vi "8 PulseGenerations.vi"(2 "PulseGen Packets":u64[](array[numeric])=[0, 0, 0, 0, 0, 0, 0, 0], 4 "8 PulseGen Chs":T1={"DO0"="Connector0/DIO4", "DO1"="Connector0/DIO5", "DO2"="Connector0/DIO6", "DO3"="Connector0/DIO7", "DO4"="Connector0/DIO12", "DO5"="Connector0/DIO13", "DO6"="Connector0/DIO14", "DO7"="Connector0/DIO15"}) -> ()   [LabVIEW 2010]
uses:
  <vilib>/eio/EIONode/EIONode.xnode
  <vilib>/rvi/eio/nirviEIOImplementation/nirviEIOImplementation.xnode
  <vilib>/rvi/eio/common/nirviEmuClasses.ctl
  <vilib>/rvi/eio/common/nirviEmuTemplateMethod_noerrors.vi
  <vilib>/NI Veristand/FPGA/NI_VS FPGA Support.lvlib
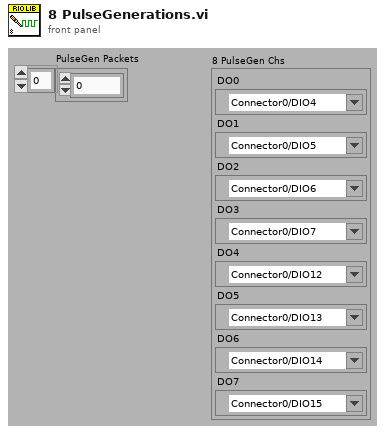
[diagram p1: front panel]
types:
  T1 = cluster{"DO0":refnum<k21>, "DO1":refnum<k21>, "DO2":refnum<k21>, "DO3":refnum<k21>, "DO4":refnum<k21>, "DO5":refnum<k21>, "DO6":refnum<k21>, "DO7":refnum<k21>}
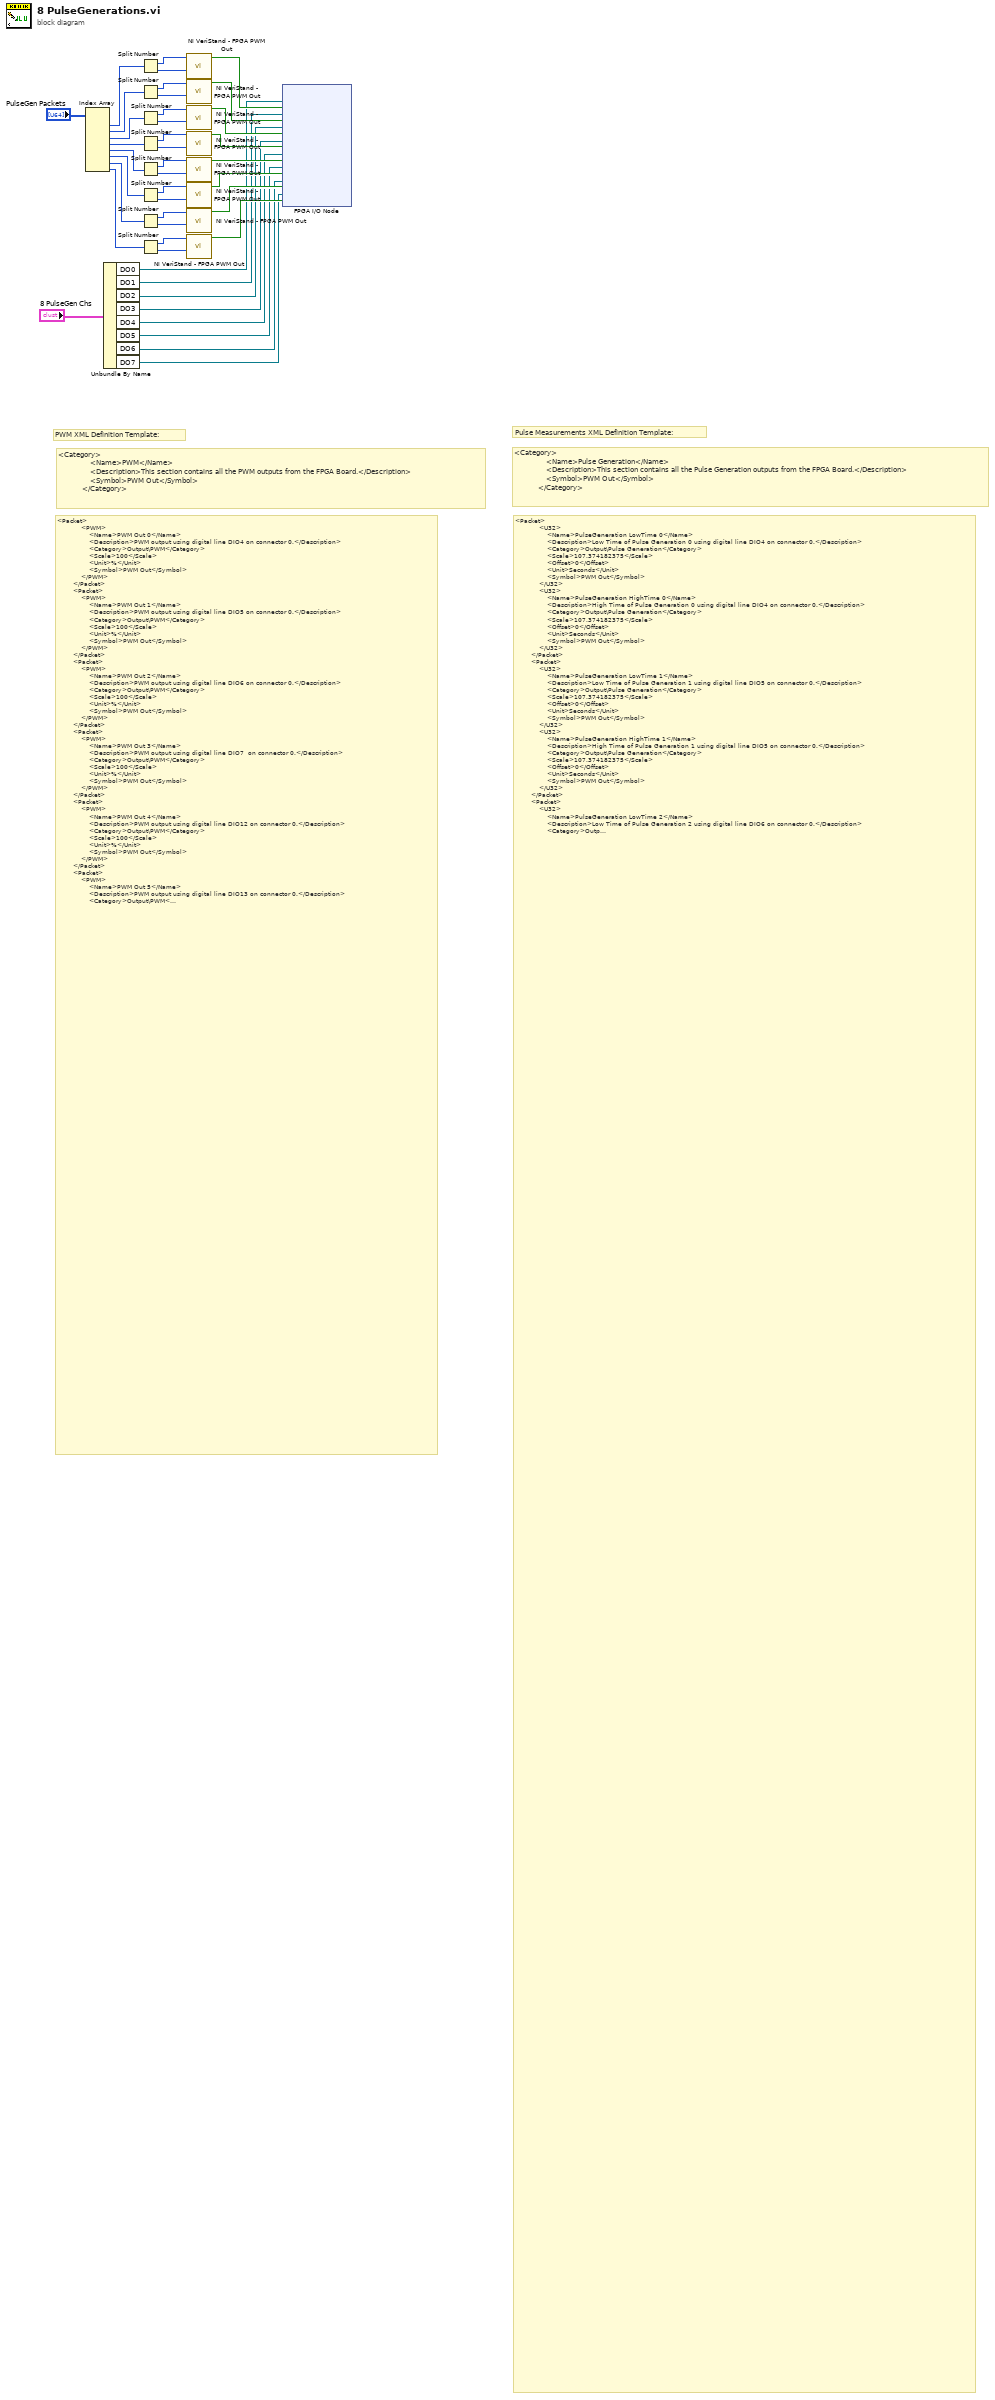
[diagram p0: block diagram]
diagram:
  # "<Category>\n                <Name>Pulse Generation</Name>\n                <Description>This section contains all the Pulse Generation outputs from the FPGA Board.</Description>\n                <Symbol>PWM Out</Symbol>\n            </Category>"
  # "<Category>\n                <Name>PWM</Name>\n                <Description>This section contains all the PWM outputs from the FPGA Board.</Description>\n                <Symbol>PWM Out</Symbol>\n            </Category>"
  # "Pulse Measurements XML Definition Template:"
  # "<Packet>\n            <U32>\n                <Name>PulseGeneration LowTime 0</Name>\n                <Description>Low Time of Pulse Generation 0 using digital line DIO4 on connector 0.</Description>\n                <Category>Output\\Pulse Generation</Category>\n                <Scale>107.374182375</Scale>\n                <Offset>0</Offset>\n                <Unit>Seconds</Unit>\n                <Symbol>PWM Out</Symbol>\n            </U32>\n            <U32>\n                <Name>PulseGeneration HighTime 0</Name>\n                <Description>High Time of Pulse Generation 0 using digital line DIO4 on connector 0.</Description>\n                <Category>Output\\Pulse Generation</Category>\n                <Scale>107.374182375</Scale>\n                <Offset>0</Offset>\n                <Unit>Seconds</Unit>\n                <Symbol>PWM Out</Symbol>\n            </U32>\n        </Packet>\n        <Packet>\n            <U32>\n                <Name>PulseGeneration LowTime 1</Name>\n                <Description>Low Time of Pulse Generation 1 using digital line DIO5 on connector 0.</Description>\n                <Category>Output\\Pulse Generation</Category>\n                <Scale>107.374182375</Scale>\n                <Offset>0</Offset>\n                <Unit>Seconds</Unit>\n                <Symbol>PWM Out</Symbol>\n            </U32>\n            <U32>\n                <Name>PulseGeneration HighTime 1</Name>\n                <Description>High Time of Pulse Generation 1 using digital line DIO5 on connector 0.</Description>\n                <Category>Output\\Pulse Generation</Category>\n                <Scale>107.374182375</Scale>\n                <Offset>0</Offset>\n                <Unit>Seconds</Unit>\n                <Symbol>PWM Out</Symbol>\n            </U32>\n        </Packet>\n        <Packet>\n            <U32>\n                <Name>PulseGeneration LowTime 2</Name>\n                <Description>Low Time of Pulse Generation 2 using digital line DIO6 on connector 0.</Description>\n                <Category>Output\\Pulse Generation</Category>\n                <Scale>107.374182375</Scale>\n                <Offset>0</Offset>\n                <Unit>Seconds</Unit>\n                <Symbol>PWM Out</Symbol>\n            </U32>\n            <U32>\n                <Name>PulseGeneration HighTime 2</Name>\n                <Description>High Time of Pulse Generation 2 using digital line DIO6 on connector 0.</Description>\n                <Category>Output\\Pulse Generation</Category>\n                <Scale>107.374182375</Scale>\n                <Offset>0</Offset>\n                <Unit>Seconds</Unit>\n                <Symbol>PWM Out</Symbol>\n            </U32>\n        </Packet>\n        <Packet>\n            <U32>\n                <Name>PulseGeneration LowTime 3</Name>\n                <Description>Low Time of Pulse Generation 3 using digital line DIO7 on connector 0.</Description>\n                <Category>Output\\Pulse Generation</Category>\n                <Scale>107.374182375</Scale>\n                <Offset>0</Offset>\n                <Unit>Seconds</Unit>\n                <Symbol>PWM Out</Symbol>\n            </U32>\n            <U32>\n                <Name>PulseGeneration HighTime 3</Name>\n                <Description>High Time of Pulse Generation 3 using digital line DIO7 on connector 0.</Description>\n                <Category>Output\\Pulse Generation</Category>\n                <Scale>107.374182375</Scale>\n                <Offset>0</Offset>\n                <Unit>Seconds</Unit>\n                <Symbol>PWM Out</Symbol>\n            </U32>\n        </Packet>\n        <Packet>\n            <U32>\n                <Name>PulseGeneration LowTime 4</Name>\n                <Description>Low Time of Pulse Generation 4 using digital line DIO12 on connector 0.</Description>\n                <Category>Output\\Pulse Generation</Category>\n                <Scale>107.374182375</Scale>\n                <Offset>0</Offset>\n                <Unit>Seconds</Unit>\n                <Symbol>PWM Out</Symbol>\n            </U32>\n            <U32>\n                <Name>PulseGeneration HighTime 4</Name>\n                <Description>High Time of Pulse Generation 4 using digital line DIO12 on connector 0.</Description>\n                <Category>Output\\Pulse Generation</Category>\n                <Scale>107.374182375</Scale>\n                <Offset>0</Offset>\n                <Unit>Seconds</Unit>\n                <Symbol>PWM Out</Symbol>\n            </U32>\n        </Packet>\n        <Packet>\n            <U32>\n                <Name>PulseGeneration LowTime 5</Name>\n                <Description>Low Time of Pulse Generation 5 using digital line DIO13 on connector 0.</Description>\n                <Category>Output\\Pulse Generation</Category>\n                <Scale>107.374182375</Scale>\n                <Offset>0</Offset>\n                <Unit>Seconds</Unit>\n                <Symbol>PWM Out</Symbol>\n            </U32>\n            <U32>\n                <Name>PulseGeneration HighTime 5</Name>\n                <Description>High Time of Pulse Generation 5 using digital line DIO13 on connector 0.</Description>\n                <Category>Output\\Pulse Generation</Category>\n                <Scale>107.374182375</Scale>\n                <Offset>0</Offset>\n                <Unit>Seconds</Unit>\n                <Symbol>PWM Out</Symbol>\n            </U32>\n        </Packet>\n        <Packet>\n            <U32>\n                <Name>PulseGeneration LowTime 6</Name>\n                <Description>Low Time of Pulse Generation 6 using digital line DIO14 on connector 0.</Description>\n                <Category>Output\\Pulse Generation</Category>\n                <Scale>107.374182375</Scale>\n                <Offset>0</Offset>\n                <Unit>Seconds</Unit>\n                <Symbol>PWM Out</Symbol>\n            </U32>\n            <U32>\n                <Name>PulseGeneration HighTime 6</Name>\n                <Description>High Time of Pulse Generation 6 using digital line DIO14 on connector 0.</Description>\n                <Category>Output\\Pulse Generation</Category>\n                <Scale>107.374182375</Scale>\n                <Offset>0</Offset>\n                <Unit>Seconds</Unit>\n                <Symbol>PWM Out</Symbol>\n            </U32>\n        </Packet>\n        <Packet>\n            <U32>\n                <Name>PulseGeneration LowTime 7</Name>\n                <Description>Low Time of Pulse Generation 7 using digital line DIO15 on connector 0.</Description>\n                <Category>Output\\Pulse Generation</Category>\n                <Scale>107.374182375</Scale>\n                <Offset>0</Offset>\n                <Unit>Seconds</Unit>\n                <Symbol>PWM Out</Symbol>\n            </U32>\n            <U32>\n                <Name>PulseGeneration HighTime 7</Name>\n                <Description>High Time of Pulse Generation 7 using digital line DIO15 on connector 0.</Description>\n                <Category>Output\\Pulse Generation</Category>\n                <Scale>107.374182375</Scale>\n                <Offset>0</Offset>\n                <Unit>Seconds</Unit>\n                <Symbol>PWM Out</Symbol>\n            </U32>\n        </Packet>"
  # "PWM XML Definition Template:"
  # "<Packet>\n            <PWM>\n                <Name>PWM Out 0</Name>\n                <Description>PWM output using digital line DIO4 on connector 0.</Description>\n                <Category>Output\\PWM</Category>\n                <Scale>100</Scale>\n                <Unit>%</Unit>\n                <Symbol>PWM Out</Symbol>\n            </PWM>\n        </Packet>\n        <Packet>\n            <PWM>\n                <Name>PWM Out 1</Name>\n                <Description>PWM output using digital line DIO5 on connector 0.</Description>\n                <Category>Output\\PWM</Category>\n                <Scale>100</Scale>\n                <Unit>%</Unit>\n                <Symbol>PWM Out</Symbol>\n            </PWM>\n        </Packet>\n        <Packet>\n            <PWM>\n                <Name>PWM Out 2</Name>\n                <Description>PWM output using digital line DIO6 on connector 0.</Description>\n                <Category>Output\\PWM</Category>\n                <Scale>100</Scale>\n                <Unit>%</Unit>\n                <Symbol>PWM Out</Symbol>\n            </PWM>\n        </Packet>\n        <Packet>\n            <PWM>\n                <Name>PWM Out 3</Name>\n                <Description>PWM output using digital line DIO7  on connector 0.</Description>\n                <Category>Output\\PWM</Category>\n                <Scale>100</Scale>\n                <Unit>%</Unit>\n                <Symbol>PWM Out</Symbol>\n            </PWM>\n        </Packet>\n        <Packet>\n            <PWM>\n                <Name>PWM Out 4</Name>\n                <Description>PWM output using digital line DIO12 on connector 0.</Description>\n                <Category>Output\\PWM</Category>\n                <Scale>100</Scale>\n                <Unit>%</Unit>\n                <Symbol>PWM Out</Symbol>\n            </PWM>\n        </Packet>\n        <Packet>\n            <PWM>\n                <Name>PWM Out 5</Name>\n                <Description>PWM output using digital line DIO13 on connector 0.</Description>\n                <Category>Output\\PWM</Category>\n                <Scale>100</Scale>\n                <Unit>%</Unit>\n                <Symbol>PWM Out</Symbol>\n            </PWM>\n        </Packet>\n        <Packet>\n            <PWM>\n                <Name>PWM Out 6</Name>\n                <Description>PWM output using digital line DIO14 on connector 0.</Description>\n                <Category>Output\\PWM</Category>\n                <Scale>100</Scale>\n                <Unit>%</Unit>\n                <Symbol>PWM Out</Symbol>\n            </PWM>\n        </Packet>\n        <Packet>\n            <PWM>\n                <Name>PWM Out 7</Name>\n                <Description>PWM output using digital line DIO15 on connector 0.</Description>\n                <Category>Output\\PWM</Category>\n                <Scale>100</Scale>\n                <Unit>%</Unit>\n                <Symbol>PWM Out</Symbol>\n            </PWM>\n        </Packet>"
  n1 = Index Array(array="PulseGen Packets") -> (element #1=w33:u64, element #2=w34:u64, element #3=w35:u64, element #4=w40:u64, element #5=w39:u64, element #6=w38:u64, element #7=w37:u64, element #8=w36:u64)  [unwired: 8 in]
  n2 = Unbundle By Name("8 PulseGen Chs") -> ("DO0"=w8:refnum<k21>, "DO1"=w7:refnum<k21>, "DO2"=w6:refnum<k21>, "DO3"=w5:refnum<k21>, "DO4"=w4:refnum<k21>, "DO5"=w3:refnum<k21>, "DO6"=w2:refnum<k21>, "DO7"=w1:refnum<k21>)
  n3 = Split Number(x=w33) -> (hi(x)=w11:u32, lo(x)=w12:u32)
  n4 = Split Number(x=w34) -> (hi(x)=w14:u32, lo(x)=w13:u32)
  n5 = Split Number(x=w35) -> (hi(x)=w15:u32, lo(x)=w16:u32)
  n6 = Split Number(x=w40) -> (hi(x)=w18:u32, lo(x)=w17:u32)
  n7 = Split Number(x=w39) -> (hi(x)=w19:u32, lo(x)=w20:u32)
  n8 = Split Number(x=w38) -> (hi(x)=w22:u32, lo(x)=w21:u32)
  n9 = Split Number(x=w37) -> (hi(x)=w23:u32, lo(x)=w24:u32)
  n10 = Split Number(x=w36) -> (hi(x)=w26:u32, lo(x)=w25:u32)
  n11 = call <vilib>:"NI VeriStand - FPGA PWM Out.vi"("_Low Time"=w12, "_High Time"=w11) -> ("Output"=w10:bool)  [unwired: 1 in, 8 out]
  n12 = call <vilib>:"NI VeriStand - FPGA PWM Out.vi"("_Low Time"=w13, "_High Time"=w14) -> ("Output"=w41:bool)  [unwired: 1 in, 8 out]
  n13 = call <vilib>:"NI VeriStand - FPGA PWM Out.vi"("_Low Time"=w16, "_High Time"=w15) -> ("Output"=w42:bool)  [unwired: 1 in, 8 out]
  n14 = call <vilib>:"NI VeriStand - FPGA PWM Out.vi"("_Low Time"=w17, "_High Time"=w18) -> ("Output"=w31:bool)  [unwired: 1 in, 8 out]
  n15 = call <vilib>:"NI VeriStand - FPGA PWM Out.vi"("_Low Time"=w20, "_High Time"=w19) -> ("Output"=w30:bool)  [unwired: 1 in, 8 out]
  n16 = call <vilib>:"NI VeriStand - FPGA PWM Out.vi"("_Low Time"=w21, "_High Time"=w22) -> ("Output"=w29:bool)  [unwired: 1 in, 8 out]
  n17 = call <vilib>:"NI VeriStand - FPGA PWM Out.vi"("_Low Time"=w24, "_High Time"=w23) -> ("Output"=w28:bool)  [unwired: 1 in, 8 out]
  n18 = call <vilib>:"NI VeriStand - FPGA PWM Out.vi"("_Low Time"=w25, "_High Time"=w26) -> ("Output"=w27:bool)  [unwired: 1 in, 8 out]
  n19 = xnode "FPGA I/O Node"("I/O Item"=w10, "I/O Item"=w41, "I/O Item"=w42, "I/O Item"=w31, "I/O Item"=w30, "I/O Item"=w29, "I/O Item"=w28, "I/O Item"=w27, "FPGA I/O In"=w8, "FPGA I/O In"=w7, "FPGA I/O In"=w6, "FPGA I/O In"=w5, "FPGA I/O In"=w4, "FPGA I/O In"=w3, "FPGA I/O In"=w2, "FPGA I/O In"=w1) -> ()  [unwired: 8 out]
